vi "SendToDatabase.vi"(8 "error in (no error)":errorcluster, 10 "Database ref":refnum<k24>, 11 "BLE Message in":refnum<class "BLE Message.lvclass">) -> (0 "error out":errorcluster)   [LabVIEW 2015, in "BLE Message.lvclass"]
uses:
  BLE Message.lvclass
  C:/Users/Bartek/Desktop/NORDIC Labview GUI/DLLs/NordicDatabaseDLL.dll
  DLLs/NordicDatabaseDLL.dll
  BLE Message.lvclass/BLE Message.ctl
  ctrls/DataBaseData.ctl
  ctrls/AccelerometerData.ctl
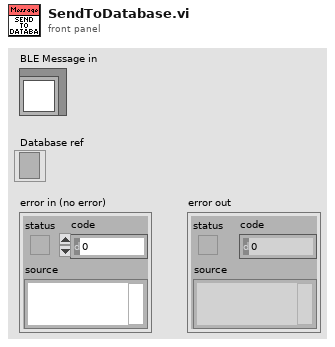
[diagram p1: front panel]
types:
  T1 = typedef "DataBaseData.ctl" = cluster{"HeartRate":u32[], "ACC data":T2[]}
  T2 = typedef "AccelerometerData.ctl" = cluster{"X":dbl, "Y":dbl, "Z":dbl}
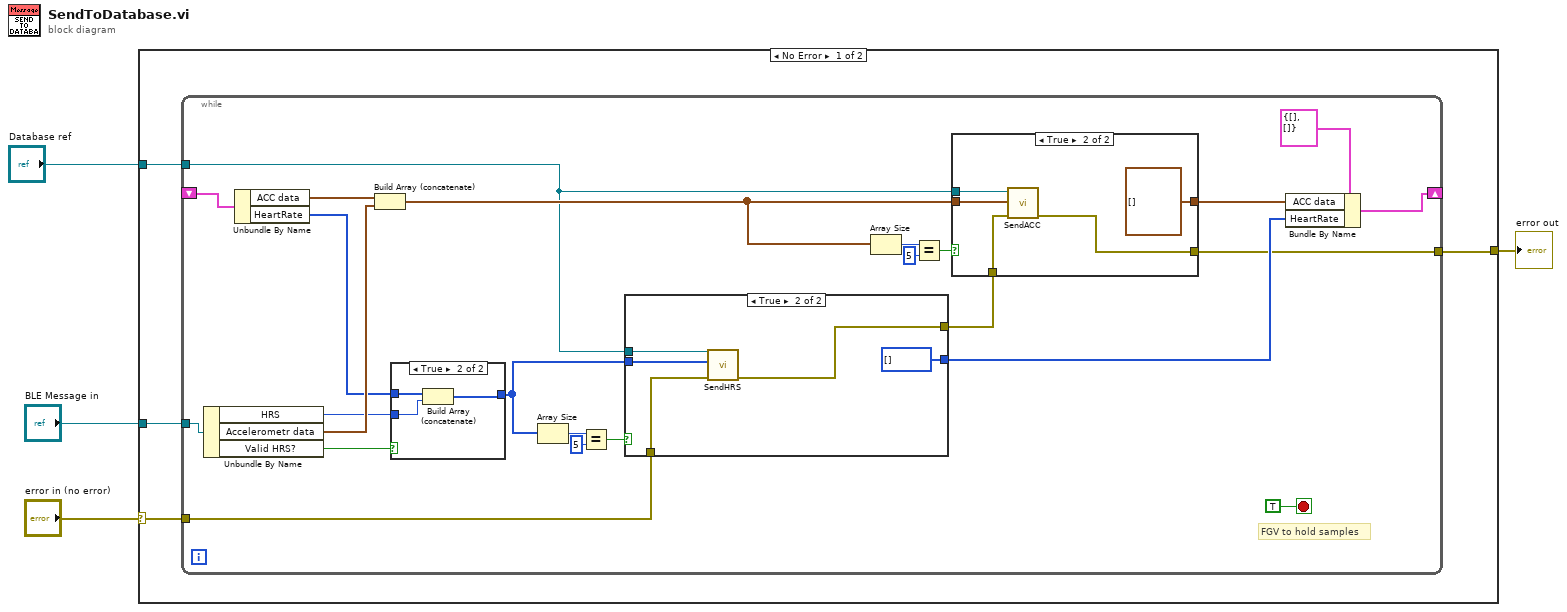
[diagram p0: block diagram]
diagram:
  n1 = case shown="No Error" "error in (no error)" {
    selector: "error in (no error)" -> [w8 w51]
    tunnel: [w5 w51] -> w3
    tunnel: "BLE Message in" -> [w7 _]
    tunnel: "Database ref" -> [w6 _]
    frame No Error {
      n2 = while {
        tunnel: w8 -> [w12]
        shift-right: [w29] -> _
        shift-left: _ -> [w28]
        tunnel: w7 -> [w31]
        tunnel: w6 -> [w13]
        tunnel: [w9] -> w5
        stop <- TRUE stop-if-true
        # "FGV to hold samples"
        n3 = Unbundle By Name(w31) -> ("HRS"=w23:u32, "Accelerometr data"=w26:T2, "Valid HRS?"=w25:bool)
        n4 = Unbundle By Name(w28) -> ("ACC data"=w27:T2[], "HeartRate"=w24:u32[])
        n5 = Build Array (concatenate)(w27, w26) -> (w19:T2[])
        n6 = case shown="True" w25 {
          tunnel: w24 -> [w47 w50]
          tunnel: w23 -> [_ w49]
          tunnel: [w47 w48] -> w15
          frame False {
          }
          frame True {
            n7 = Build Array (concatenate)(w50, w49) -> (w48:u32[])
          }
        }
        n8 = Array Size(array=w15) -> (size(s)=w16:i32)
        n9 = Equal?(x=w16, y=5) -> (x = y?=w11:bool)
        n10 = case shown="True" w11 {
          tunnel: w15 -> [w34 w39]
          tunnel: [w34 u32[] [] ("HeartRate")] -> w14
          tunnel: w13 -> [_ w38]
          tunnel: w12 -> [w33 w37]
          tunnel: [w33 w35] -> w10
          frame False {
          }
          frame True {
            n11 = call "SendHRS.vi"("error in (no error)"=w37, "HRS data"=w39, "Database ref"=w38) -> ("error out"=w35:errorcluster)  [unwired: 8 in]
          }
        }
        n12 = Array Size(array=w19) -> (size(s)=w22:i32)
        n13 = Equal?(x=w22, y=5) -> (x = y?=w21:bool)
        n14 = case shown="True" w21 {
          tunnel: w19 -> [w41 w46]
          tunnel: [w41 T2[] []] -> w18
          tunnel: w13 -> [_ w45]
          tunnel: w10 -> [w40 w43]
          tunnel: [w40 w42] -> w9
          frame False {
          }
          frame True {
            n15 = call "SendACC.vi"("error in (no error)"=w43, "appended array"=w46, "Database ref"=w45) -> ("error out"=w42:errorcluster)  [unwired: 8 in]
          }
        }
        n16 = Bundle By Name(cluster=T1 {"HeartRate"=[], "ACC data"=[]} ("Data"), "ACC data"=w18, "HeartRate"=w14) -> (w29:T1)
      }
    }
    frame Error {
    }
  }
  "error out" <- w3
